vi "trash_Plugin Subpanel Initialization Wrapper.vi"(8 "error in (no error)":errorcluster, 11 "CIF_UI in":refnum<class "CIF_UI.lvclass">) -> (0 "error out":errorcluster, 3 "CIF_UI out":refnum<class "CIF_UI.lvclass">)   [LabVIEW 2021]
uses:
  CIF_UI.lvclass
  Typedef/Class Data for SubPanel.ctl
  <vilib>/gRPC/LabVIEW gRPC Library/Shared/grpcId.ctl
  Typedef/Core UI References.ctl
  Typedef/Channel Connection.ctl
  Typedef/New Plugin.ctl
  Typedef/Run Listen Button.ctl
  Typedef/CIF_Manager_UI_Tab.ctl
  Typedef/SubPanel Events.ctl
  Typedef/New Connection Event Data.ctl
  Typedef/New Connection Plugin Event Data.ctl
  CIF_UI.lvclass/CIF_UI.ctl
  Plugins/Template/Grpc/Template_wrapper/TemplateWrapper.lvlib
  <vilib>/gRPC/LabVIEW gRPC Library/grpc-lvsupport-release.lvlib
panel:
  out "Event Registration Refnum":refnum<event-registration>
  in  "Calling VI":refnum<vi>
  in  "Class Data for SubPanel":T1
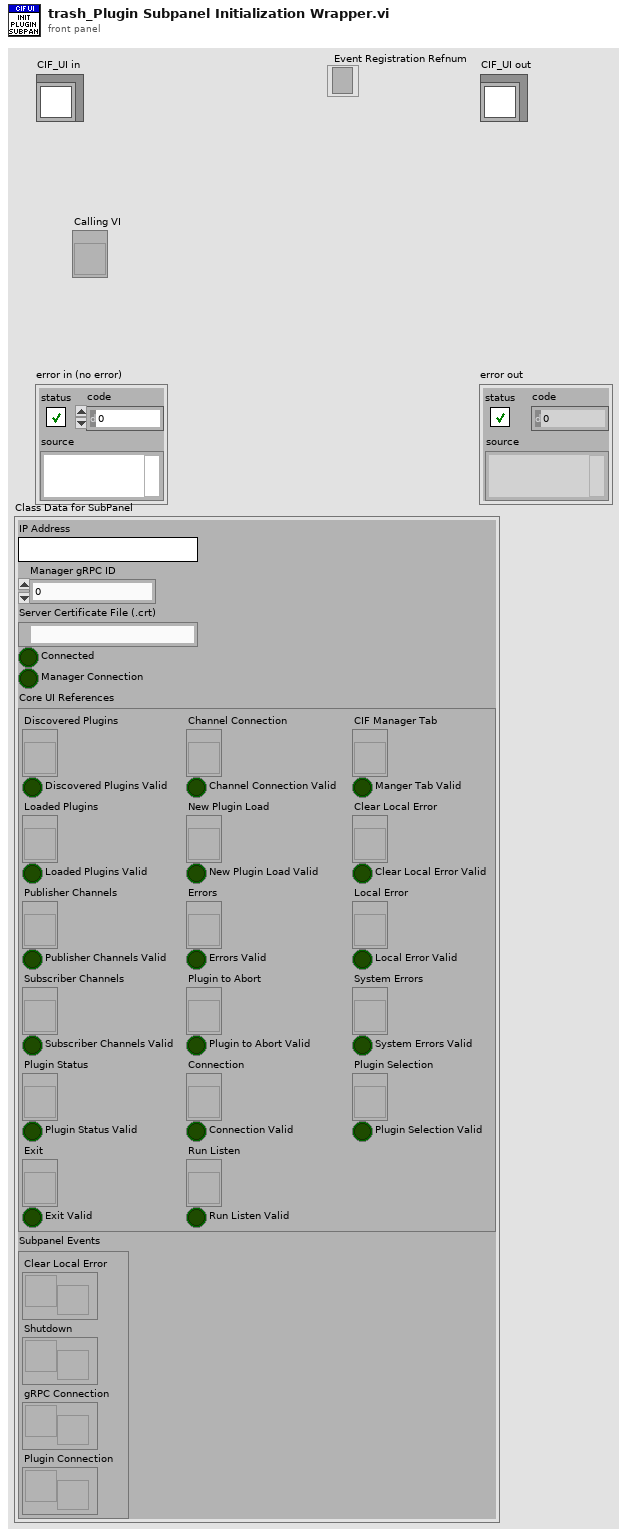
[diagram p1: front panel]
types:
  T1 = typedef "CIF_UI.lvclass/Class Data for SubPanel.ctl" = cluster{"IP Address":string, "Manager gRPC ID":T2, "Server Certificate File (.crt)":path, "Connected":bool, "Manager Connection":bool, "Core UI References":T3, "Subpanel Events":T4}
  T2 = typedef "grpc-lvsupport-release.lvlib/grpcId.ctl" = u64
  T3 = typedef "CIF_UI.lvclass/Core UI References.ctl" = cluster{"Discovered Plugins":refnum<vi>, "Discovered Plugins Valid":bool, "Loaded Plugins":refnum<vi>, "Loaded Plugins Valid":bool, "Publisher Channels":refnum<vi>, "Publisher Channels Valid":bool, "Subscriber Channels":refnum<vi>, "Subscriber Channels Valid":bool, "Plugin Status":refnum<vi>, "Plugin Status Valid":bool, "Channel Connection":refnum<vi>, "Channel Connection Valid":bool, "New Plugin Load":refnum<vi>, "New Plugin Load Valid":bool, "Errors":refnum<vi>, "Errors Valid":bool, "Plugin to Abort":refnum<vi>, "Plugin to Abort Valid":bool, "Connection":refnum<vi>, "Connection Valid":bool, "Exit":refnum<vi>, "Exit Valid":bool, "Run Listen":refnum<vi>, "Run Listen Valid":bool, "CIF Manager Tab":refnum<vi>, "Manger Tab Valid":bool, "Clear Local Error":refnum<vi>, "Clear Local Error Valid":bool, "Local Error":refnum<vi>, "Local Error Valid":bool, "System Errors":refnum<vi>, "System Errors Valid":bool, "Plugin Selection":refnum<vi>, "Plugin Selection Valid":bool}
  T4 = typedef "CIF_UI.lvclass/SubPanel Events.ctl" = cluster{"Clear Local Error":refnum<user-event>, "Shutdown":refnum<user-event>, "gRPC Connection":refnum<user-event>, "Plugin Connection":refnum<user-event>}
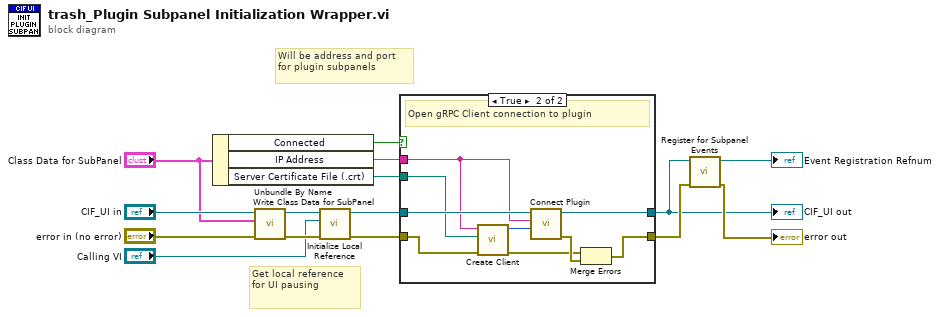
[diagram p0: block diagram]
diagram:
  # "Will be address and port for plugin subpanels"
  # "Get local reference for UI pausing"
  n1 = Unbundle By Name("Class Data for SubPanel") -> ("Connected"=w10:bool, "IP Address"=w9:string, "Server Certificate File (.crt)"=w8:path)
  n2 = call "Write Class Data for SubPanel.vi"("error in (no error)"="error in (no error)", "Class Data for SubPanel"="Class Data for SubPanel", "CIF_UI in"="CIF_UI in") -> ("error out"=w14:errorcluster, "CIF_UI out"=w15:refnum<class "CIF_UI.lvclass">)  [unwired: 7 in]
  n3 = call "Initialize Local Reference.vi"("error in (no error)"=w14, "This VI"="Calling VI", "CIF_UI in"=w15) -> ("error out"=w12:errorcluster, "CIF_UI out"=w13:refnum<class "CIF_UI.lvclass">)  [unwired: 7 in]
  n4 = case shown="True" w10 {
    tunnel: [w16 w26] -> w11
    tunnel: [w17 w24] -> w3
    tunnel: w13 -> [w17 w23]
    tunnel: w12 -> [w16 w22]
    tunnel: w9 -> [_ w19]
    tunnel: w8 -> [_ w18]
    frame False {
    }
    frame True {
      # "Open gRPC Client connection to plugin"
      n5 = call "Create Client.vi"("error in"=w22, "Server Certificate File (.crt)"=w18, "address"=w19) -> ("error out"=w21:errorcluster, "gRPC ID Out"=w20:T2)  [unwired: 7 in]
      n6 = call "Connect Plugin.vi"("gRPC ID"=w20, "Address"=w19, "CIF_UI in"=w23) -> ("error out"=w25:errorcluster, "CIF_UI out"=w24:refnum<class "CIF_UI.lvclass">)  [unwired: 7 in]
      n7 = Merge Errors(w21, w25) -> (w26:errorcluster)
    }
  }
  "CIF_UI out" <- w3
  n8 = call "Register for Subpanel Events.vi"("error in (no error)"=w11, "CIF_UI in"=w3) -> ("error out"=→"error out":errorcluster, "Event Registration Refnum"=→"Event Registration Refnum":refnum<event-registration>)  [unwired: 8 in]
